vi "HARVESTOR w ELEVATOR  SUBVI.vi"   [LabVIEW 2011]
types:
  T1 = cluster{"Digital Input [1-16][0]":bool, "Digital Input [1-16][1]":bool, "Digital Input [1-16][2]":bool, "Digital Input [1-16][3]":bool, "Digital Input [1-16][4]":bool, "Digital Input [1-16][5]":bool, "Digital Input [1-16][6]":bool, "Digital Input [1-16][7]":bool, "Digital Input [1-16][8]":bool}
  T2 = cluster{"Digital Input [1-16][0]":bool, "Digital Input [1-16][1]":bool, "Digital Input [1-16][2]":bool, "Digital Input [1-16][3]":bool, "Digital Input [1-16][4]":bool, "Digital Input [1-16][5]":bool, "Digital Input [1-16][6]":bool, "Digital Input [1-16][7]":bool, "Digital Input [1-16][8]":bool, "Digital Input [1-16][9]":bool, "Digital Input [1-16][10]":bool, "Digital Input [1-16][11]":bool, "Digital Input [1-16][12]":bool, "Digital Input [1-16][13]":bool, "Digital Input [1-16][14]":bool, "Digital Input [1-16][15]":bool}
  T3 = typedef "WPI_MotorControlDeviceRef.ctl" = cluster{"DeviceStatus":errorcluster, "Type":enum16{"PWM", "CAN"}, "PWM":cluster{"Digital Module":T4, "PWM Channel":T5, "DeadBand":T6}, "CAN":cluster{"Device Number":u8, "Control Mode":T7, "Semaphore":T8, "Max Vout":dbl}, "Invert":bool, "TransformRef":T9, "InvTransformRef":T9}
  T4 = typedef "FPGA_TypedefDigitalModule.ctl" = enum16{"Digital Module 1", "Digital Module 2"}
  T5 = typedef "FPGA_DIOPWMChannel.ctl" = enum8{"PWM 1", "PWM 2", "PWM 3", "PWM 4", "PWM 5", "PWM 6", "PWM 7", "PWM 8", "PWM 9", "PWM 10", "Invalid"}
  T6 = typedef "WPI_PWMDeadband.ctl" = cluster{"Name":string, "maxPositivePwm":i32, "minPositivePwm":i32, "centerPwm":i32, "maxNegativePwm":i32, "minNegativePwm":i32, "angularRange":u16}
  T7 = typedef "WPI_CANJaguar_ControlMode.ctl" = enum8{"Percent VBus", "Current", "Speed", "Position", "Voltage"}
  T8 = typedef "Semaphore RefNum" = refnum<k1>
  T9 = typedef "WPI_PWMTransform_ConPane.ctl" = refnum<vi>
  T10 = typedef "WPI_DigitalInputDevRef.ctl" = cluster{"DevStatus":errorcluster, "DIO Channel":T11, "Digital Module":T4}
  T11 = typedef "FPGA_DIOChannel.ctl" = enum8{"DIO 1", "DIO 2", "DIO 3", "DIO 4", "DIO 5", "DIO 6", "DIO 7", "DIO 8", "DIO 9", "DIO 10", "DIO 11", "DIO 12", "DIO 13", "DIO 14", "Invalid"}
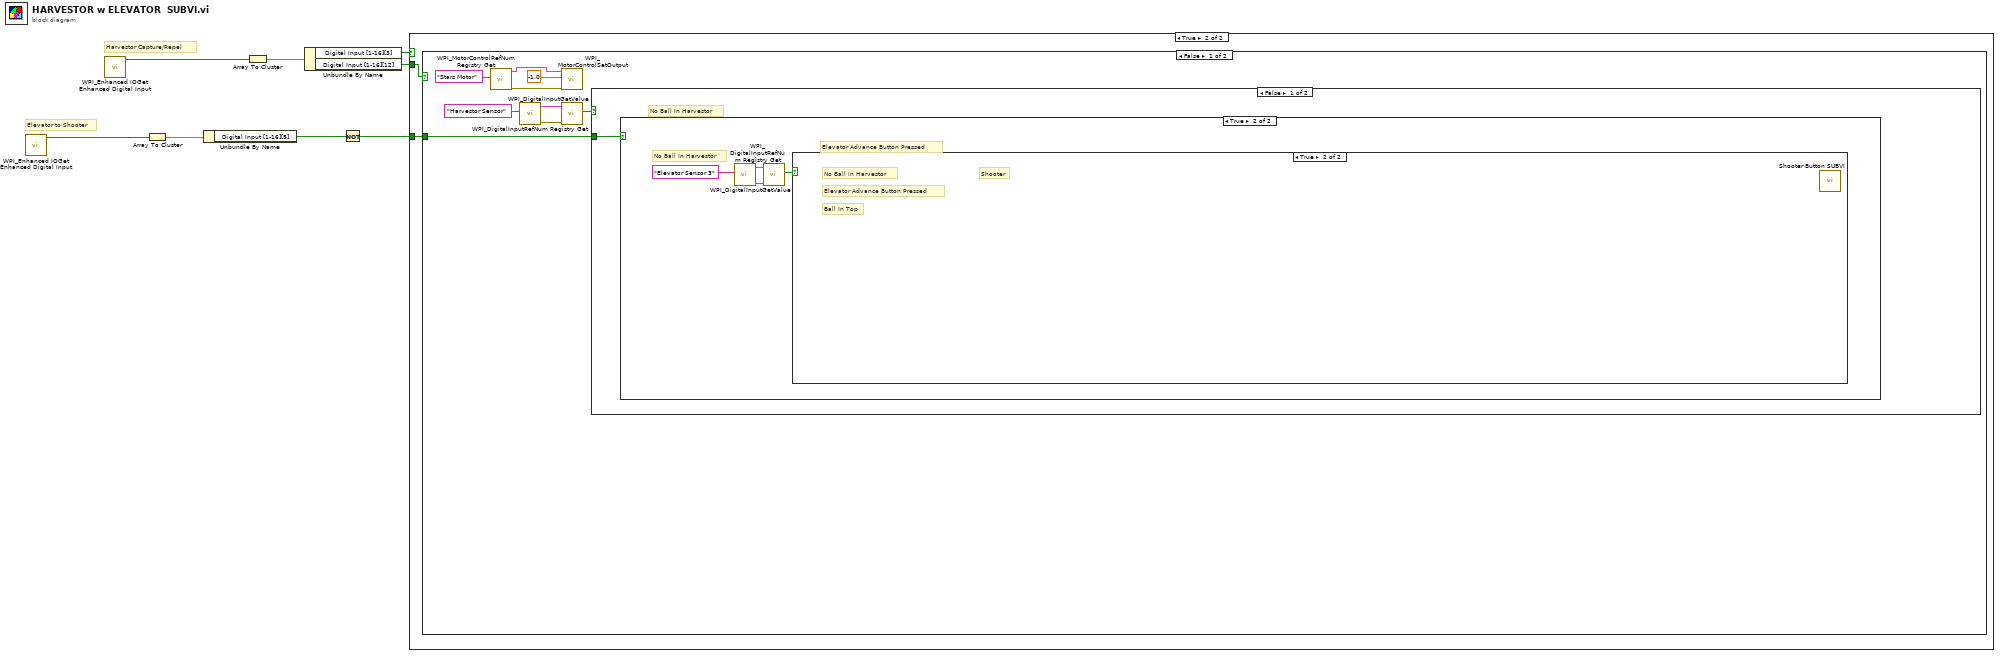
[diagram p0: block diagram]
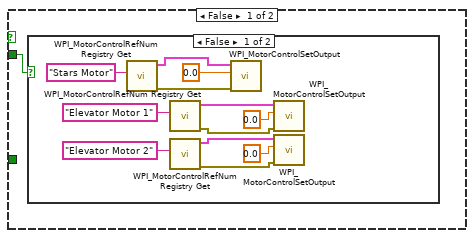
[diagram p2: hidden frame]
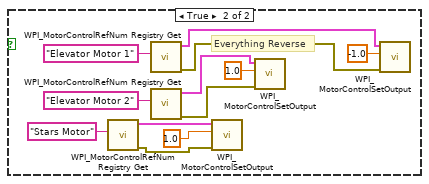
[diagram p3: hidden frame]
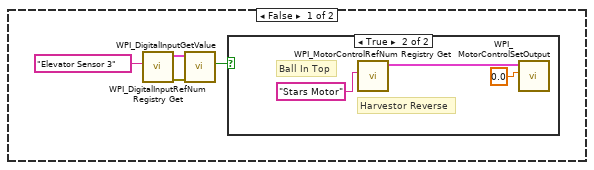
[diagram p4: hidden frame]
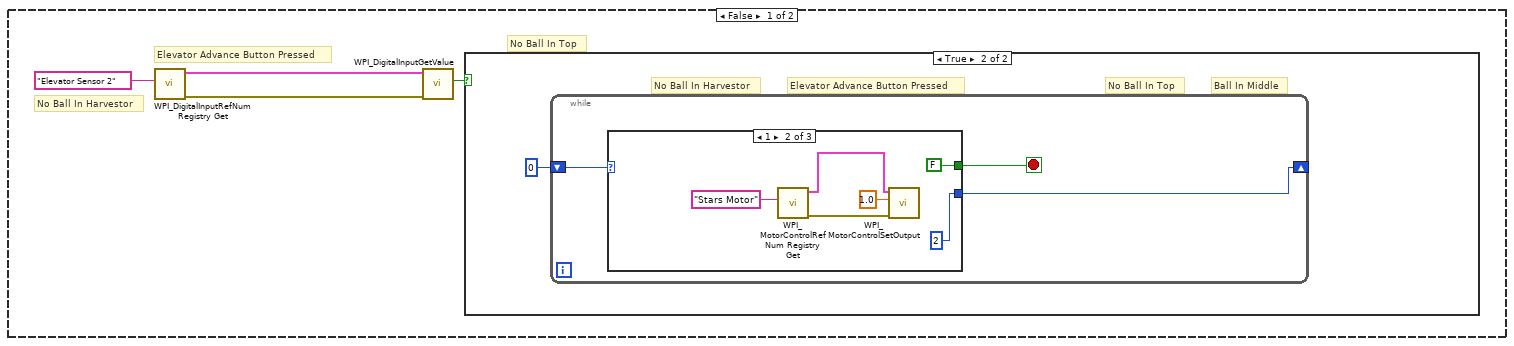
[diagram p6: hidden frame]
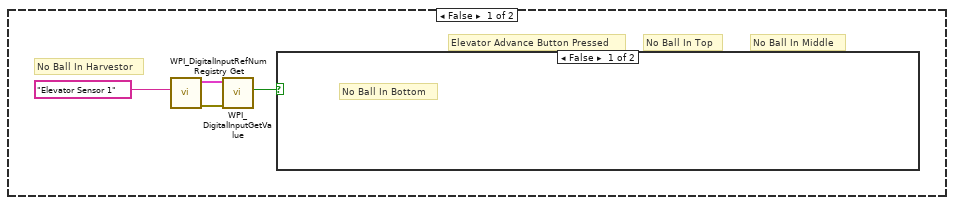
[diagram p7: hidden frame]
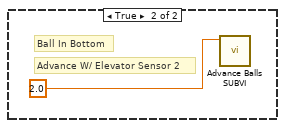
[diagram p8: hidden frame]
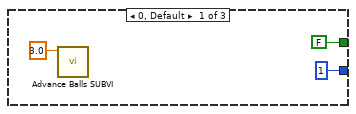
[diagram p9: hidden frame]
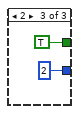
[diagram p10: hidden frame]
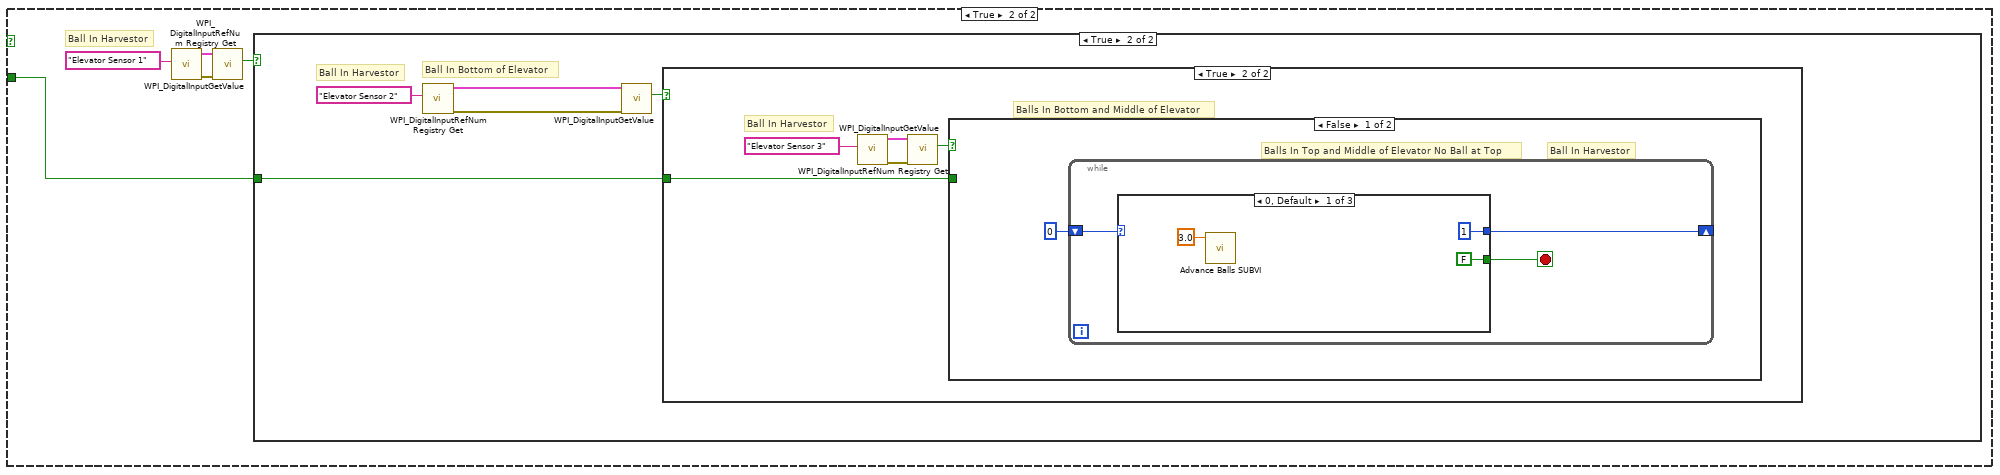
[diagram p11: hidden frame]
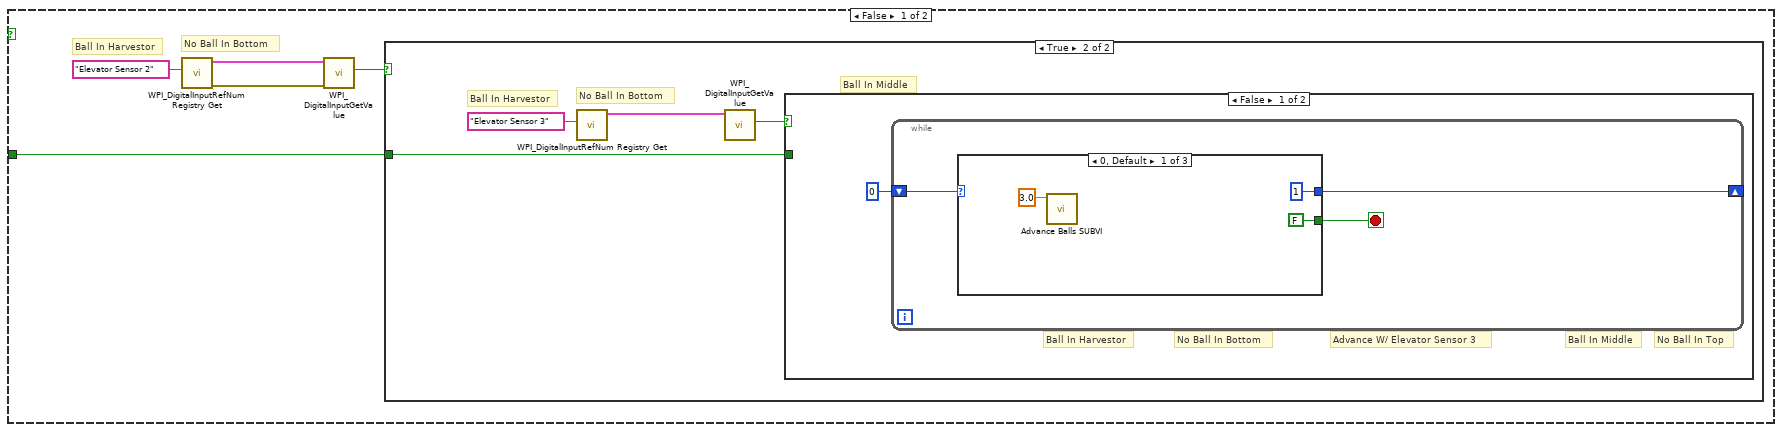
[diagram p12: hidden frame]
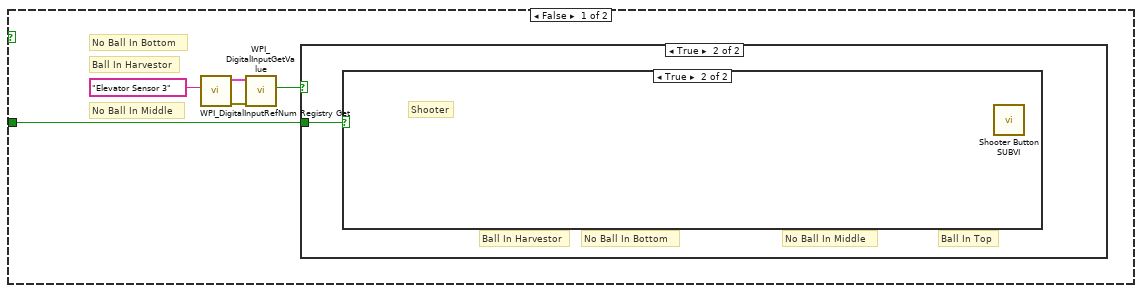
[diagram p13: hidden frame]
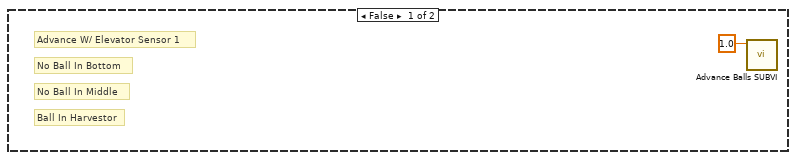
[diagram p14: hidden frame]
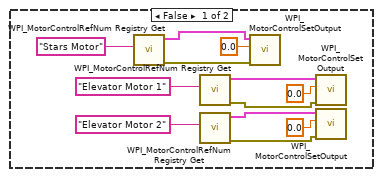
[diagram p15: hidden frame]
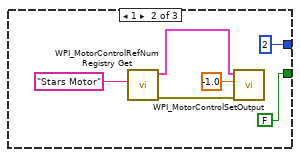
[diagram p16: hidden frame]
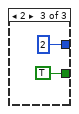
[diagram p17: hidden frame]
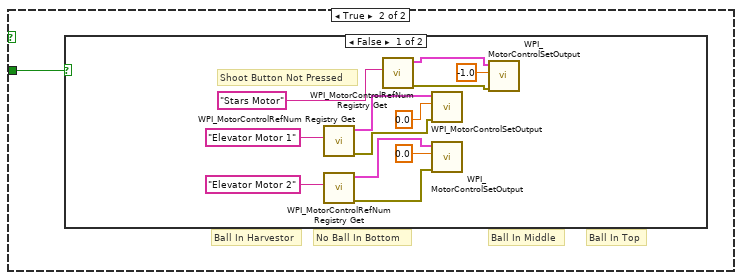
[diagram p18: hidden frame]
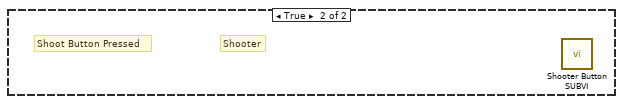
[diagram p19: hidden frame]
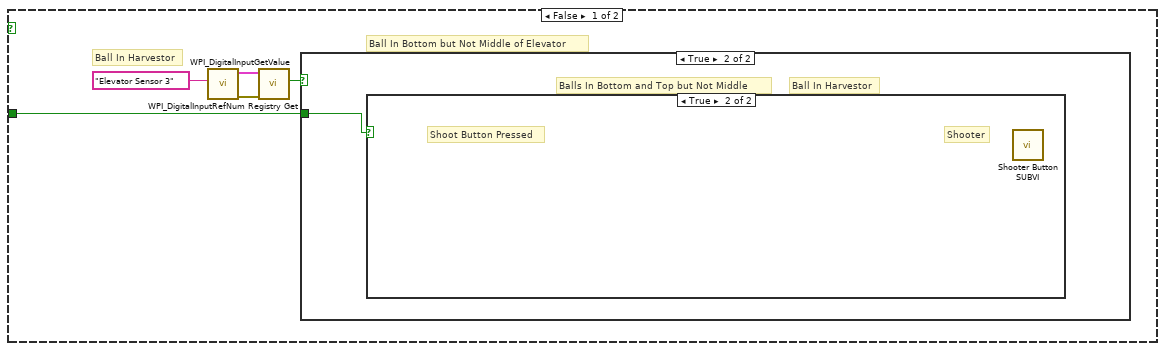
[diagram p20: hidden frame]
diagram:
  # "Elevator to Shooter"
  # "Harvestor Capture/Repel"
  n1 = call <vilib>:"WPI_Enhanced IOGet Enhanced Digital Input.vi"() -> ("Digital Input [1-16]"=w5:bool[])  [unwired: 10 in, 1 out]
  n2 = call <vilib>:"WPI_Enhanced IOGet Enhanced Digital Input.vi"() -> ("Digital Input [1-16]"=w1:bool[])  [unwired: 10 in, 1 out]
  n3 = Array To Cluster(array=w5) -> (cluster=w6:T1)
  n4 = Unbundle By Name(w6) -> ("Digital Input [1-16][5]"=w7:bool)
  n5 = Array To Cluster(array=w1) -> (cluster=w2:T2)
  n6 = Unbundle By Name(w2) -> ("Digital Input [1-16][3]"=w3:bool, "Digital Input [1-16][12]"=w4:bool)
  n7 = Not(x=w7) -> (.not. x?=w8:bool)
  n8 = case shown="True" w3 {
    tunnel: w4 -> [w9 w35]
    tunnel: w8 -> [_ w34]
    frame False {
      n9 = case shown="False" w9 {
        frame False {
          n10 = call <vilib>:"WPI_MotorControlRefNum Registry Get.vi"("refnum name"="Stars Motor") -> ("error out"=w10:errorcluster, "MotorControlDevRef"=w11:T3)  [unwired: 9 in]
          n11 = call <vilib>:"WPI_MotorControlRefNum Registry Get.vi"("refnum name"="Elevator Motor 1") -> ("error out"=w17:errorcluster, "MotorControlDevRef"=w18:T3)  [unwired: 9 in]
          n12 = call <vilib>:"WPI_MotorControlRefNum Registry Get.vi"("refnum name"="Elevator Motor 2") -> ("error out"=w14:errorcluster, "MotorControlDevRef"=w15:T3)  [unwired: 9 in]
          n13 = call <vilib>:"WPI_MotorControlSetOutput.vi"("error in (no error)"=w10, "Output"=0.0, "MotorControlDevRef"=w11) -> ()  [unwired: 7 in, 2 out]
          n14 = call <vilib>:"WPI_MotorControlSetOutput.vi"("error in (no error)"=w17, "Output"=0.0, "MotorControlDevRef"=w18) -> ()  [unwired: 7 in, 2 out]
          n15 = call <vilib>:"WPI_MotorControlSetOutput.vi"("error in (no error)"=w14, "Output"=0.0, "MotorControlDevRef"=w15) -> ()  [unwired: 7 in, 2 out]
        }
        frame True {
          # "Everything Reverse"
          n16 = call <vilib>:"WPI_MotorControlRefNum Registry Get.vi"("refnum name"="Stars Motor") -> ("error out"=w22:errorcluster, "MotorControlDevRef"=w23:T3)  [unwired: 9 in]
          n17 = call <vilib>:"WPI_MotorControlRefNum Registry Get.vi"("refnum name"="Elevator Motor 1") -> ("error out"=w29:errorcluster, "MotorControlDevRef"=w30:T3)  [unwired: 9 in]
          n18 = call <vilib>:"WPI_MotorControlRefNum Registry Get.vi"("refnum name"="Elevator Motor 2") -> ("error out"=w26:errorcluster, "MotorControlDevRef"=w27:T3)  [unwired: 9 in]
          n19 = call <vilib>:"WPI_MotorControlSetOutput.vi"("error in (no error)"=w22, "Output"=1.0, "MotorControlDevRef"=w23) -> ()  [unwired: 7 in, 2 out]
          n20 = call <vilib>:"WPI_MotorControlSetOutput.vi"("error in (no error)"=w26, "Output"=1.0, "MotorControlDevRef"=w27) -> ()  [unwired: 7 in, 2 out]
          n21 = call <vilib>:"WPI_MotorControlSetOutput.vi"("error in (no error)"=w29, "Output"=-1.0, "MotorControlDevRef"=w30) -> ()  [unwired: 7 in, 2 out]
        }
      }
    }
    frame True {
      n22 = case shown="False" w35 {
        tunnel: w34 -> [w36 w203]
        frame False {
          n23 = call <vilib>:"WPI_MotorControlRefNum Registry Get.vi"("refnum name"="Stars Motor") -> ("error out"=w37:errorcluster, "MotorControlDevRef"=w38:T3)  [unwired: 9 in]
          n24 = call <vilib>:"WPI_DigitalInputRefNum Registry Get.vi"("refnum name"="Harvestor Sensor") -> ("error out"=w41:errorcluster, "DigitalInputDevRef"=w42:T10)  [unwired: 9 in]
          n25 = call <vilib>:"WPI_MotorControlSetOutput.vi"("error in (no error)"=w37, "Output"=-1.0, "MotorControlDevRef"=w38) -> ()  [unwired: 7 in, 2 out]
          n26 = call <vilib>:"WPI_DigitalInputGetValue.vi"("error in (no error)"=w41, "DigitalInputDevRef"=w42) -> ("Value"=w44:bool)  [unwired: 7 in, 2 out]
          n27 = case shown="False" w44 {
            tunnel: w36 -> [w45 w82]
            frame False {
              # "No Ball In Harvestor"
              n28 = case shown="True" w45 {
                frame False {
                  n29 = call <vilib>:"WPI_DigitalInputRefNum Registry Get.vi"("refnum name"="Elevator Sensor 3") -> ("error out"=w47:errorcluster, "DigitalInputDevRef"=w48:T10)  [unwired: 9 in]
                  n30 = call <vilib>:"WPI_DigitalInputGetValue.vi"("error in (no error)"=w47, "DigitalInputDevRef"=w48) -> ("Value"=w46:bool)  [unwired: 7 in, 2 out]
                  n31 = case shown="True" w46 {
                    frame False {
                    }
                    frame True {
                      # "Harvestor Reverse"
                      # "Ball In Top"
                      n32 = call <vilib>:"WPI_MotorControlRefNum Registry Get.vi"("refnum name"="Stars Motor") -> ("MotorControlDevRef"=w50:T3)  [unwired: 9 in, 1 out]
                      n33 = call <vilib>:"WPI_MotorControlSetOutput.vi"("Output"=0.0, "MotorControlDevRef"=w50) -> ()  [unwired: 8 in, 2 out]
                    }
                  }
                }
                frame True {
                  # "No Ball In Harvestor"
                  # "Elevator Advance Button Pressed"
                  n34 = call <vilib>:"WPI_DigitalInputRefNum Registry Get.vi"("refnum name"="Elevator Sensor 3") -> ("error out"=w55:errorcluster, "DigitalInputDevRef"=w56:T10)  [unwired: 9 in]
                  n35 = call <vilib>:"WPI_DigitalInputGetValue.vi"("error in (no error)"=w55, "DigitalInputDevRef"=w56) -> ("Value"=w54:bool)  [unwired: 7 in, 2 out]
                  n36 = case shown="True" w54 {
                    frame False {
                      # "No Ball In Top"
                      # "No Ball In Harvestor"
                      # "Elevator Advance Button Pressed"
                      n37 = call <vilib>:"WPI_DigitalInputRefNum Registry Get.vi"("refnum name"="Elevator Sensor 2") -> ("error out"=w59:errorcluster, "DigitalInputDevRef"=w60:T10)  [unwired: 9 in]
                      n38 = call <vilib>:"WPI_DigitalInputGetValue.vi"("error in (no error)"=w59, "DigitalInputDevRef"=w60) -> ("Value"=w57:bool)  [unwired: 7 in, 2 out]
                      n39 = case shown="True" w57 {
                        frame False {
                          # "No Ball In Middle"
                          # "No Ball In Top"
                          # "No Ball In Harvestor"
                          # "Elevator Advance Button Pressed"
                          n40 = call <vilib>:"WPI_DigitalInputRefNum Registry Get.vi"("refnum name"="Elevator Sensor 1") -> ("error out"=w62:errorcluster, "DigitalInputDevRef"=w63:T10)  [unwired: 9 in]
                          n41 = call <vilib>:"WPI_DigitalInputGetValue.vi"("error in (no error)"=w62, "DigitalInputDevRef"=w63) -> ("Value"=w61:bool)  [unwired: 7 in, 2 out]
                          n42 = case shown="False" w61 {
                            frame False {
                              # "No Ball In Bottom"
                            }
                            frame True {
                              # "Ball In Bottom"
                              # "Advance W/ Elevator Sensor 2"
                              n43 = call "Advance Balls SUBVI.vi"("Numeric"=2.0) -> ()  [unwired: 11 in]
                            }
                          }
                        }
                        frame True {
                          # "Ball In Middle"
                          # "No Ball In Top"
                          # "No Ball In Harvestor"
                          # "Elevator Advance Button Pressed"
                          n44 = while {
                            shift-right: [w68] -> _
                            shift-left: 0 -> [w69]
                            stop <- w67 stop-if-true
                            n45 = case shown="1" w69 {
                              tunnel: [1 2 2] -> w68
                              tunnel: [FALSE FALSE TRUE] -> w67
                              frame 0, Default {
                                n46 = call "Advance Balls SUBVI.vi"("Numeric"=3.0) -> ()  [unwired: 11 in]
                              }
                              frame 1 {
                                n47 = call <vilib>:"WPI_MotorControlRefNum Registry Get.vi"("refnum name"="Stars Motor") -> ("error out"=w77:errorcluster, "MotorControlDevRef"=w76:T3)  [unwired: 9 in]
                                n48 = call <vilib>:"WPI_MotorControlSetOutput.vi"("error in (no error)"=w77, "Output"=1.0, "MotorControlDevRef"=w76) -> ()  [unwired: 7 in, 2 out]
                              }
                              frame 2 {
                              }
                            }
                          }
                        }
                      }
                    }
                    frame True {
                      # "Ball In Top"
                      # "No Ball In Harvestor"
                      # "Elevator Advance Button Pressed"
                      # "Shooter"
                      n49 = call "Shooter Button SUBVI.vi"() -> ()  [unwired: 12 in]
                    }
                  }
                }
              }
            }
            frame True {
              # "Ball In Harvestor"
              n50 = call <vilib>:"WPI_DigitalInputRefNum Registry Get.vi"("refnum name"="Elevator Sensor 1") -> ("error out"=w83:errorcluster, "DigitalInputDevRef"=w84:T10)  [unwired: 9 in]
              n51 = call <vilib>:"WPI_DigitalInputGetValue.vi"("error in (no error)"=w83, "DigitalInputDevRef"=w84) -> ("Value"=w81:bool)  [unwired: 7 in, 2 out]
              n52 = case shown="True" w81 {
                tunnel: w82 -> [w87 w144]
                frame False {
                  # "No Ball In Bottom"
                  # "Ball In Harvestor"
                  n53 = call <vilib>:"WPI_DigitalInputRefNum Registry Get.vi"("refnum name"="Elevator Sensor 2") -> ("error out"=w89:errorcluster, "DigitalInputDevRef"=w90:T10)  [unwired: 9 in]
                  n54 = call <vilib>:"WPI_DigitalInputGetValue.vi"("error in (no error)"=w89, "DigitalInputDevRef"=w90) -> ("Value"=w88:bool)  [unwired: 7 in, 2 out]
                  n55 = case shown="True" w88 {
                    tunnel: w87 -> [w92 w112]
                    frame False {
                      # "No Ball In Middle"
                      # "No Ball In Bottom"
                      # "Ball In Harvestor"
                      n56 = call <vilib>:"WPI_DigitalInputRefNum Registry Get.vi"("refnum name"="Elevator Sensor 3") -> ("error out"=w94:errorcluster, "DigitalInputDevRef"=w95:T10)  [unwired: 9 in]
                      n57 = call <vilib>:"WPI_DigitalInputGetValue.vi"("error in (no error)"=w94, "DigitalInputDevRef"=w95) -> ("Value"=w93:bool)  [unwired: 7 in, 2 out]
                      n58 = case shown="True" w93 {
                        tunnel: w92 -> [_ w97]
                        frame False {
                          # "No Ball In Middle"
                          # "No Ball In Bottom"
                          # "Ball In Harvestor"
                          # "Advance W/ Elevator Sensor 1"
                          n59 = call "Advance Balls SUBVI.vi"("Numeric"=1.0) -> ()  [unwired: 11 in]
                        }
                        frame True {
                          # "Ball In Top"
                          # "No Ball In Middle"
                          # "No Ball In Bottom"
                          # "Ball In Harvestor"
                          n60 = case shown="True" w97 {
                            frame False {
                              n61 = call <vilib>:"WPI_MotorControlRefNum Registry Get.vi"("refnum name"="Stars Motor") -> ("error out"=w98:errorcluster, "MotorControlDevRef"=w99:T3)  [unwired: 9 in]
                              n62 = call <vilib>:"WPI_MotorControlRefNum Registry Get.vi"("refnum name"="Elevator Motor 1") -> ("error out"=w105:errorcluster, "MotorControlDevRef"=w106:T3)  [unwired: 9 in]
                              n63 = call <vilib>:"WPI_MotorControlRefNum Registry Get.vi"("refnum name"="Elevator Motor 2") -> ("error out"=w102:errorcluster, "MotorControlDevRef"=w103:T3)  [unwired: 9 in]
                              n64 = call <vilib>:"WPI_MotorControlSetOutput.vi"("error in (no error)"=w98, "Output"=0.0, "MotorControlDevRef"=w99) -> ()  [unwired: 7 in, 2 out]
                              n65 = call <vilib>:"WPI_MotorControlSetOutput.vi"("error in (no error)"=w105, "Output"=0.0, "MotorControlDevRef"=w106) -> ()  [unwired: 7 in, 2 out]
                              n66 = call <vilib>:"WPI_MotorControlSetOutput.vi"("error in (no error)"=w102, "Output"=0.0, "MotorControlDevRef"=w103) -> ()  [unwired: 7 in, 2 out]
                            }
                            frame True {
                              # "Shooter"
                              n67 = call "Shooter Button SUBVI.vi"() -> ()  [unwired: 12 in]
                            }
                          }
                        }
                      }
                    }
                    frame True {
                      # "Ball In Middle"
                      # "No Ball In Bottom"
                      # "Ball In Harvestor"
                      n68 = call <vilib>:"WPI_DigitalInputRefNum Registry Get.vi"("refnum name"="Elevator Sensor 3") -> ("DigitalInputDevRef"=w113:T10)  [unwired: 9 in, 1 out]
                      n69 = call <vilib>:"WPI_DigitalInputGetValue.vi"("DigitalInputDevRef"=w113) -> ("Value"=w110:bool)  [unwired: 8 in, 2 out]
                      n70 = case shown="False" w110 {
                        tunnel: w112 -> [_ w129]
                        frame False {
                          # "No Ball In Top"
                          # "Ball In Middle"
                          # "No Ball In Bottom"
                          # "Ball In Harvestor"
                          # "Advance W/ Elevator Sensor 3"
                          n71 = while {
                            shift-right: [w116] -> _
                            shift-left: 0 -> [w117]
                            stop <- w115 stop-if-true
                            n72 = case shown="0, Default" w117 {
                              tunnel: [1 2 2] -> w116
                              tunnel: [FALSE FALSE TRUE] -> w115
                              frame 0, Default {
                                n73 = call "Advance Balls SUBVI.vi"("Numeric"=3.0) -> ()  [unwired: 11 in]
                              }
                              frame 1 {
                                n74 = call <vilib>:"WPI_MotorControlRefNum Registry Get.vi"("refnum name"="Stars Motor") -> ("error out"=w125:errorcluster, "MotorControlDevRef"=w124:T3)  [unwired: 9 in]
                                n75 = call <vilib>:"WPI_MotorControlSetOutput.vi"("error in (no error)"=w125, "Output"=-1.0, "MotorControlDevRef"=w124) -> ()  [unwired: 7 in, 2 out]
                              }
                              frame 2 {
                              }
                            }
                          }
                        }
                        frame True {
                          # "Ball In Top"
                          # "Ball In Middle"
                          # "No Ball In Bottom"
                          # "Ball In Harvestor"
                          n76 = case shown="False" w129 {
                            frame False {
                              # "Shoot Button Not Pressed"
                              n77 = call <vilib>:"WPI_MotorControlRefNum Registry Get.vi"("refnum name"="Elevator Motor 1") -> ("error out"=w137:errorcluster, "MotorControlDevRef"=w138:T3)  [unwired: 9 in]
                              n78 = call <vilib>:"WPI_MotorControlRefNum Registry Get.vi"("refnum name"="Elevator Motor 2") -> ("error out"=w134:errorcluster, "MotorControlDevRef"=w135:T3)  [unwired: 9 in]
                              n79 = call <vilib>:"WPI_MotorControlRefNum Registry Get.vi"("refnum name"="Stars Motor") -> ("error out"=w130:errorcluster, "MotorControlDevRef"=w131:T3)  [unwired: 9 in]
                              n80 = call <vilib>:"WPI_MotorControlSetOutput.vi"("error in (no error)"=w137, "Output"=0.0, "MotorControlDevRef"=w138) -> ()  [unwired: 7 in, 2 out]
                              n81 = call <vilib>:"WPI_MotorControlSetOutput.vi"("error in (no error)"=w134, "Output"=0.0, "MotorControlDevRef"=w135) -> ()  [unwired: 7 in, 2 out]
                              n82 = call <vilib>:"WPI_MotorControlSetOutput.vi"("error in (no error)"=w130, "Output"=-1.0, "MotorControlDevRef"=w131) -> ()  [unwired: 7 in, 2 out]
                            }
                            frame True {
                              # "Shoot Button Pressed"
                              # "Shooter"
                              n83 = call "Shooter Button SUBVI.vi"() -> ()  [unwired: 12 in]
                            }
                          }
                        }
                      }
                    }
                  }
                }
                frame True {
                  # "Ball In Harvestor"
                  # "Ball In Bottom of Elevator"
                  n84 = call <vilib>:"WPI_DigitalInputRefNum Registry Get.vi"("refnum name"="Elevator Sensor 2") -> ("error out"=w145:errorcluster, "DigitalInputDevRef"=w146:T10)  [unwired: 9 in]
                  n85 = call <vilib>:"WPI_DigitalInputGetValue.vi"("error in (no error)"=w145, "DigitalInputDevRef"=w146) -> ("Value"=w142:bool)  [unwired: 7 in, 2 out]
                  n86 = case shown="True" w142 {
                    tunnel: w144 -> [w148 w167]
                    frame False {
                      # "Ball In Harvestor"
                      # "Ball In Bottom but Not Middle of Elevator"
                      n87 = call <vilib>:"WPI_DigitalInputRefNum Registry Get.vi"("refnum name"="Elevator Sensor 3") -> ("error out"=w150:errorcluster, "DigitalInputDevRef"=w151:T10)  [unwired: 9 in]
                      n88 = call <vilib>:"WPI_DigitalInputGetValue.vi"("error in (no error)"=w150, "DigitalInputDevRef"=w151) -> ("Value"=w149:bool)  [unwired: 7 in, 2 out]
                      n89 = case shown="True" w149 {
                        tunnel: w148 -> [_ w153]
                        frame False {
                          # "Advance W/ Elevator Sensor 2"
                          n90 = call "Advance Balls SUBVI.vi"("Numeric"=2.0) -> ()  [unwired: 11 in]
                        }
                        frame True {
                          # "Ball In Harvestor"
                          # "Balls In Bottom and Top but Not Middle"
                          n91 = case shown="True" w153 {
                            frame False {
                              # "Ball In Harvestor"
                              # "Balls In Bottom and Top Shoot Button Not Pressed"
                              n92 = call <vilib>:"WPI_MotorControlRefNum Registry Get.vi"("refnum name"="Stars Motor") -> ("error out"=w154:errorcluster, "MotorControlDevRef"=w155:T3)  [unwired: 9 in]
                              n93 = call <vilib>:"WPI_MotorControlRefNum Registry Get.vi"("refnum name"="Elevator Motor 2") -> ("error out"=w158:errorcluster, "MotorControlDevRef"=w159:T3)  [unwired: 9 in]
                              n94 = call <vilib>:"WPI_MotorControlRefNum Registry Get.vi"("refnum name"="Elevator Motor 1") -> ("error out"=w161:errorcluster, "MotorControlDevRef"=w162:T3)  [unwired: 9 in]
                              n95 = call <vilib>:"WPI_MotorControlSetOutput.vi"("error in (no error)"=w158, "Output"=0.0, "MotorControlDevRef"=w159) -> ()  [unwired: 7 in, 2 out]
                              n96 = call <vilib>:"WPI_MotorControlSetOutput.vi"("error in (no error)"=w161, "Output"=0.0, "MotorControlDevRef"=w162) -> ()  [unwired: 7 in, 2 out]
                              n97 = call <vilib>:"WPI_MotorControlSetOutput.vi"("error in (no error)"=w154, "Output"=0.0, "MotorControlDevRef"=w155) -> ()  [unwired: 7 in, 2 out]
                            }
                            frame True {
                              # "Shoot Button Pressed"
                              # "Shooter"
                              n98 = call "Shooter Button SUBVI.vi"() -> ()  [unwired: 12 in]
                            }
                          }
                        }
                      }
                    }
                    frame True {
                      # "Ball In Harvestor"
                      # "Balls In Bottom and Middle of Elevator"
                      n99 = call <vilib>:"WPI_DigitalInputRefNum Registry Get.vi"("refnum name"="Elevator Sensor 3") -> ("error out"=w169:errorcluster, "DigitalInputDevRef"=w170:T10)  [unwired: 9 in]
                      n100 = call <vilib>:"WPI_DigitalInputGetValue.vi"("error in (no error)"=w169, "DigitalInputDevRef"=w170) -> ("Value"=w168:bool)  [unwired: 7 in, 2 out]
                      n101 = case shown="False" w168 {
                        tunnel: w167 -> [_ w186]
                        frame False {
                          # "Ball In Harvestor"
                          # "Balls In Top and Middle of Elevator No Ball at Top"
                          n102 = while {
                            shift-right: [w173] -> _
                            shift-left: 0 -> [w174]
                            stop <- w172 stop-if-true
                            n103 = case shown="0, Default" w174 {
                              tunnel: [1 2 2] -> w173
                              tunnel: [FALSE FALSE TRUE] -> w172
                              frame 0, Default {
                                n104 = call "Advance Balls SUBVI.vi"("Numeric"=3.0) -> ()  [unwired: 11 in]
                              }
                              frame 1 {
                                n105 = call <vilib>:"WPI_MotorControlRefNum Registry Get.vi"("refnum name"="Stars Motor") -> ("error out"=w182:errorcluster, "MotorControlDevRef"=w181:T3)  [unwired: 9 in]
                                n106 = call <vilib>:"WPI_MotorControlSetOutput.vi"("error in (no error)"=w182, "Output"=-1.0, "MotorControlDevRef"=w181) -> ()  [unwired: 7 in, 2 out]
                              }
                              frame 2 {
                              }
                            }
                          }
                        }
                        frame True {
                          # "3 Balls In Elevator"
                          n107 = case shown="False" w186 {
                            frame False {
                              # "3 Balls In Elevator But Shoot Button Is Not Pressed"
                              n108 = call <vilib>:"WPI_MotorControlRefNum Registry Get.vi"("refnum name"="Stars Motor") -> ("error out"=w187:errorcluster, "MotorControlDevRef"=w188:T3)  [unwired: 9 in]
                              n109 = call <vilib>:"WPI_MotorControlRefNum Registry Get.vi"("refnum name"="Elevator Motor 1") -> ("error out"=w194:errorcluster, "MotorControlDevRef"=w195:T3)  [unwired: 9 in]
                              n110 = call <vilib>:"WPI_MotorControlRefNum Registry Get.vi"("refnum name"="Elevator Motor 2") -> ("error out"=w191:errorcluster, "MotorControlDevRef"=w192:T3)  [unwired: 9 in]
                              n111 = call <vilib>:"WPI_MotorControlSetOutput.vi"("error in (no error)"=w194, "Output"=0.0, "MotorControlDevRef"=w195) -> ()  [unwired: 7 in, 2 out]
                              n112 = call <vilib>:"WPI_MotorControlSetOutput.vi"("error in (no error)"=w191, "Output"=0.0, "MotorControlDevRef"=w192) -> ()  [unwired: 7 in, 2 out]
                              n113 = call <vilib>:"WPI_MotorControlSetOutput.vi"("error in (no error)"=w187, "Output"=0.0, "MotorControlDevRef"=w188) -> ()  [unwired: 7 in, 2 out]
                            }
                            frame True {
                              # "Shoot Button Is Pressed"
                              # "Shooter"
                              n114 = call "Shooter Button SUBVI.vi"() -> ()  [unwired: 12 in]
                            }
                          }
                        }
                      }
                    }
                  }
                }
              }
            }
          }
        }
        frame True {
          n115 = case shown="False" w203 {
            frame False {
              n116 = call <vilib>:"WPI_DigitalInputRefNum Registry Get.vi"("refnum name"="Elevator Sensor 3") -> ("error out"=w225:errorcluster, "DigitalInputDevRef"=w226:T10)  [unwired: 9 in]
              n117 = call <vilib>:"WPI_DigitalInputGetValue.vi"("error in (no error)"=w225, "DigitalInputDevRef"=w226) -> ("Value"=w224:bool)  [unwired: 7 in, 2 out]
              n118 = case shown="True" w224 {
                frame False {
                  # "If Elevator Advance Button Is Pressed"
                  # "Harvestor Switch Off"
                  n119 = call <vilib>:"WPI_MotorControlRefNum Registry Get.vi"("refnum name"="Stars Motor") -> ("error out"=w231:errorcluster, "MotorControlDevRef"=w228:T3)  [unwired: 9 in]
                  n120 = call <vilib>:"WPI_MotorControlSetOutput.vi"("error in (no error)"=w231, "Output"=0.0, "MotorControlDevRef"=w228) -> ()  [unwired: 7 in, 2 out]
                }
                frame True {
                  # "Harvestor Reverse"
                  # "Ball In Top"
                  n121 = call <vilib>:"WPI_MotorControlRefNum Registry Get.vi"("refnum name"="Stars Motor") -> ("error out"=w232:errorcluster, "MotorControlDevRef"=w233:T3)  [unwired: 9 in]
                  n122 = call <vilib>:"WPI_MotorControlSetOutput.vi"("error in (no error)"=w232, "Output"=0.0, "MotorControlDevRef"=w233) -> ()  [unwired: 7 in, 2 out]
                }
              }
            }
            frame True {
              # "No Ball In Harvestor"
              # "Elevator Advance Button Pressed"
              n123 = call <vilib>:"WPI_DigitalInputRefNum Registry Get.vi"("refnum name"="Elevator Sensor 3") -> ("error out"=w238:errorcluster, "DigitalInputDevRef"=w239:T10)  [unwired: 9 in]
              n124 = call <vilib>:"WPI_DigitalInputGetValue.vi"("error in (no error)"=w238, "DigitalInputDevRef"=w239) -> ("Value"=w237:bool)  [unwired: 7 in, 2 out]
              n125 = case shown="True" w237 {
                frame False {
                  # "No Ball In Top"
                  # "No Ball In Harvestor"
                  # "Elevator Advance Button Pressed"
                  n126 = call <vilib>:"WPI_DigitalInputRefNum Registry Get.vi"("refnum name"="Elevator Sensor 2") -> ("error out"=w242:errorcluster, "DigitalInputDevRef"=w243:T10)  [unwired: 9 in]
                  n127 = call <vilib>:"WPI_DigitalInputGetValue.vi"("error in (no error)"=w242, "DigitalInputDevRef"=w243) -> ("Value"=w240:bool)  [unwired: 7 in, 2 out]
                  n128 = case shown="True" w240 {
                    frame False {
                      # "No Ball In Middle"
                      # "No Ball In Top"
                      # "No Ball In Harvestor"
                      # "Elevator Advance Button Pressed"
                      n129 = call <vilib>:"WPI_DigitalInputRefNum Registry Get.vi"("refnum name"="Elevator Sensor 1") -> ("error out"=w245:errorcluster, "DigitalInputDevRef"=w246:T10)  [unwired: 9 in]
                      n130 = call <vilib>:"WPI_DigitalInputGetValue.vi"("error in (no error)"=w245, "DigitalInputDevRef"=w246) -> ("Value"=w244:bool)  [unwired: 7 in, 2 out]
                      n131 = case shown="True" w244 {
                        frame False {
                          # "No Ball In Bottom"
                          n132 = call <vilib>:"WPI_DigitalInputRefNum Registry Get.vi"("refnum name"="Harvestor Sensor") -> ("error out"=w249:errorcluster, "DigitalInputDevRef"=w250:T10)  [unwired: 9 in]
                          n133 = call <vilib>:"WPI_DigitalInputGetValue.vi"("error in (no error)"=w249, "DigitalInputDevRef"=w250) -> ("Value"=w248:bool)  [unwired: 7 in, 2 out]
                          n134 = case shown="True" w248 {
                            frame False {
                            }
                            frame True {
                              n135 = call "Advance Balls SUBVI.vi"("Numeric"=1.0) -> ()  [unwired: 11 in]
                            }
                          }
                        }
                        frame True {
                          # "Ball In Bottom"
                          # "Advance W/ Elevator Sensor 2"
                          n136 = call "Advance Balls SUBVI.vi"("Numeric"=2.0) -> ()  [unwired: 11 in]
                        }
                      }
                    }
                    frame True {
                      # "Ball In Middle"
                      # "No Ball In Top"
                      # "No Ball In Harvestor"
                      # "Elevator Advance Button Pressed"
                      n137 = while {
                        shift-right: [w256] -> _
                        shift-left: 0 -> [w257]
                        stop <- w255 stop-if-true
                        n138 = case shown="0, Default" w257 {
                          tunnel: [1 2 2] -> w256
                          tunnel: [FALSE FALSE TRUE] -> w255
                          frame 0, Default {
                            n139 = call "Advance Balls SUBVI.vi"("Numeric"=3.0) -> ()  [unwired: 11 in]
                          }
                          frame 1 {
                            n140 = call <vilib>:"WPI_MotorControlRefNum Registry Get.vi"("refnum name"="Stars Motor") -> ("error out"=w265:errorcluster, "MotorControlDevRef"=w264:T3)  [unwired: 9 in]
                            n141 = call <vilib>:"WPI_MotorControlSetOutput.vi"("error in (no error)"=w265, "Output"=1.0, "MotorControlDevRef"=w264) -> ()  [unwired: 7 in, 2 out]
                          }
                          frame 2 {
                          }
                        }
                      }
                    }
                  }
                }
                frame True {
                  # "Ball In Top"
                  # "No Ball In Harvestor"
                  # "Elevator Advance Button Pressed"
                  # "Shooter"
                }
              }
            }
          }
          n142 = call <vilib>:"WPI_DigitalInputRefNum Registry Get.vi"("refnum name"="Harvestor Sensor") -> ("error out"=w201:errorcluster, "DigitalInputDevRef"=w202:T10)  [unwired: 9 in]
          n143 = call <vilib>:"WPI_DigitalInputGetValue.vi"("error in (no error)"=w201, "DigitalInputDevRef"=w202) -> ("Value"=w200:bool)  [unwired: 7 in, 2 out]
          n144 = case shown="True" w200 {
            frame False {
              n145 = call <vilib>:"WPI_DigitalInputRefNum Registry Get.vi"("refnum name"="Elevator Sensor 1") -> ("error out"=w207:errorcluster, "DigitalInputDevRef"=w206:T10)  [unwired: 9 in]
              n146 = call <vilib>:"WPI_DigitalInputGetValue.vi"("error in (no error)"=w207, "DigitalInputDevRef"=w206) -> ("Value"=w204:bool)  [unwired: 7 in, 2 out]
              n147 = case shown="True" w204 {
                frame False {
                  # "Elevator Button"
                  n148 = call <vilib>:"WPI_DigitalInputRefNum Registry Get.vi"("refnum name"="Elevator Sensor 2") -> ("error out"=w211:errorcluster, "DigitalInputDevRef"=w210:T10)  [unwired: 9 in]
                  n149 = call <vilib>:"WPI_DigitalInputGetValue.vi"("error in (no error)"=w211, "DigitalInputDevRef"=w210) -> ("Value"=w208:bool)  [unwired: 7 in, 2 out]
                  n150 = case shown="True" w208 {
                    frame False {
                      n151 = call <vilib>:"WPI_DigitalInputRefNum Registry Get.vi"("refnum name"="Elevator Sensor 3") -> ("error out"=w215:errorcluster, "DigitalInputDevRef"=w214:T10)  [unwired: 9 in]
                      n152 = call <vilib>:"WPI_DigitalInputGetValue.vi"("error in (no error)"=w215, "DigitalInputDevRef"=w214) -> ("Value"=w212:bool)  [unwired: 7 in, 2 out]
                      n153 = case shown="True" w212 {
                        frame False {
                          n154 = call <vilib>:"WPI_MotorControlRefNum Registry Get.vi"("refnum name"="Elevator Motor 1") -> ("error out"=w220:errorcluster, "MotorControlDevRef"=w221:T3)  [unwired: 9 in]
                          n155 = call <vilib>:"WPI_MotorControlRefNum Registry Get.vi"("refnum name"="Elevator Motor 2") -> ("error out"=w216:errorcluster, "MotorControlDevRef"=w217:T3)  [unwired: 9 in]
                          n156 = call <vilib>:"WPI_MotorControlSetOutput.vi"("error in (no error)"=w220, "Output"=0.0, "MotorControlDevRef"=w221) -> ()  [unwired: 7 in, 2 out]
                          n157 = call <vilib>:"WPI_MotorControlSetOutput.vi"("error in (no error)"=w216, "Output"=0.0, "MotorControlDevRef"=w217) -> ()  [unwired: 7 in, 2 out]
                        }
                        frame True {
                        }
                      }
                    }
                    frame True {
                    }
                  }
                }
                frame True {
                }
              }
            }
            frame True {
            }
          }
        }
      }
    }
  }
